vi "Com_SECS Equipment _Stream_S7F1.vi"(8 "error in":errorcluster, 11 "S7F1 Setting":T1) -> (0 "error out":errorcluster, 3 "SECS Packet":T2)   [LabVIEW 2016]
uses:
  Data Def/Com_SECS Equipment _SECS Packet.ctl
  Data Def/Com_SECS Equipment _Message Type.ctl
  Data Def/Com_SECS Equipment _Protocol Type.ctl
  Data Def/Com_SECS Equipment _Stream Type.ctl
  Data Def/Com_SECS Equipment _Build Message Setting.ctl
  Data Message/Com_SECS Equipment _Data Message_List.vi
  Data Message/Com_SECS Equipment _Data Message_ASCII.vi
  Data Message/Com_SECS Equipment _Data Message_U4.vi
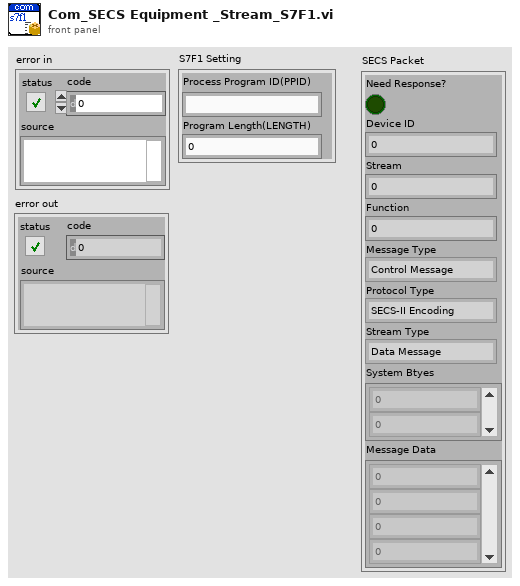
[diagram p1: front panel]
types:
  T1 = cluster{"Process Program ID(PPID)":string, "Program Length(LENGTH)":u32}
  T2 = typedef "Com_SECS Equipment _SECS Packet.ctl" = cluster{"Need Response?":bool, "Device ID":u16, "Stream":u8, "Function":u8, "Message Type":T3, "Protocol Type":T4, "Stream Type":T5, "System Btyes":u8[], "Message Data":u8[]}
  T3 = typedef "Com_SECS Equipment _Message Type.ctl" = enum16{"Control Message", "Data Message"}
  T4 = typedef "Com_SECS Equipment _Protocol Type.ctl" = enum16{"SECS-II Encoding", "Reserved"}
  T5 = typedef "Com_SECS Equipment _Stream Type.ctl" = enum16{"Data Message", "Select.req", "Select.rsp", "Deselect.req", "Deselect.rsp", "Linktest.req", "Linktest.rsp", "Reject.req", "Separate.req", "Reserve"}
  T6 = typedef "Com_SECS Equipment _Build Message Setting.ctl" = cluster{"Stream":u8, "Function":u8, "Need Response?":bool}
  T7 = typedef "Com_SECS Equipment _Message Data.ctl" = cluster{"Index":i32, "Data Item Format":T8, "Format Code":T9, "Parent Index":i32, "Child Index":i32[], "Data":variant}
  T8 = typedef "Com_SECS Equipment _Data Item Format.ctl" = enum16{"Data Type", "Value"}
  T9 = typedef "Com_SECS Equipment _Format Code.ctl" = enum16{"L", "A", "B", "Boolean", "J", "I1", "I2", "I4", "I8", "U1", "U2", "U4", "U8", "F4", "F8", "Char"}
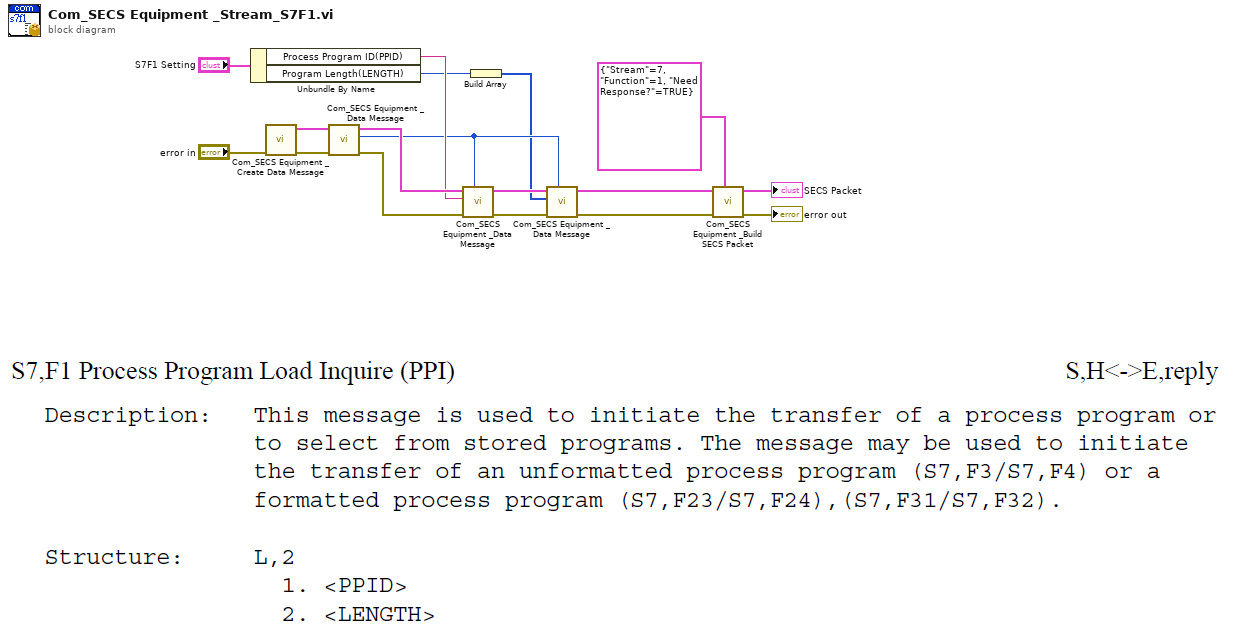
[diagram p0: block diagram]
diagram:
  n1 = Unbundle By Name("S7F1 Setting") -> ("Process Program ID(PPID)"=w8:string, "Program Length(LENGTH)"=w4:u32)
  n2 = call "Com_SECS Equipment _Create Data Message.vi"("error in"="error in") -> ("error out"=w12:errorcluster, "Message Data"=w13:T7[])  [unwired: 9 in]
  n3 = call-poly "Com_SECS Equipment _Data Message.vi"("error in"=w12, "Message Data In"=w13) -> ("error out"=w11:errorcluster, "Index"=w5:i32, "Message Data Out"=w10:T7[])  [unwired: 7 in]
  n4 = call-poly "Com_SECS Equipment _Data Message.vi"("Parent Index"=w5, "error in"=w11, "Data"=w8, "Message Data In"=w10) -> ("error out"=w7:errorcluster, "Message Data Out"=w6:T7[])  [unwired: 6 in]
  n5 = Build Array(w4) -> (w3:u32[])
  n6 = call-poly "Com_SECS Equipment _Data Message.vi"("Parent Index"=w5, "error in"=w7, "Data"=w3, "Message Data In"=w6) -> ("error out"=w1:errorcluster, "Message Data Out"=w2:T7[])  [unwired: 6 in]
  n7 = call "Com_SECS Equipment _Build SECS Packet.vi"("Build Message Setting"=T6 {"Stream"=7, "Function"=1, "Need Response?"=TRUE}, "error in"=w1, "Message Data"=w2) -> ("error out"=→"error out":errorcluster, "SECS Packet"=→"SECS Packet":T2)  [unwired: 7 in]
